vi "State of measurements func global.vi"(6 "Operation":T1(ring)=enum."Get", 9 "Active?":bool, 10 "Instruments in":refnum<class "Device.lvclass">[](array[class]), 11 "Measurement settings in":T4={"Measurements active"=FALSE, "Instruments"=[], "Save data settings"={"Save data"=TRUE, "Data Root Path"=path "", "File Prefix"="", "File Format"=enum."ASCII", "Save column names"=TRUE, "File Comments"="<Description of the current file>", "User/Prj"="<User Name/Project Description>"}, "Start time"=0}) -> (3 "Measurement settings out":T4={"Measurements active"=FALSE, "Instruments"=[], "Save data settings"={"Save data"=TRUE, "Data Root Path"=path "", "File Prefix"="", "File Format"=enum."ASCII", "Save column names"=TRUE, "File Comments"="<Description of the current file>", "User/Prj"="<User Name/Project Description>"}, "Start time"=0})   [LabVIEW 2015]
uses:
  Device/Device.lvclass
  File/Controls/Save data settings.ctl
  File/Controls/File formats.ctl
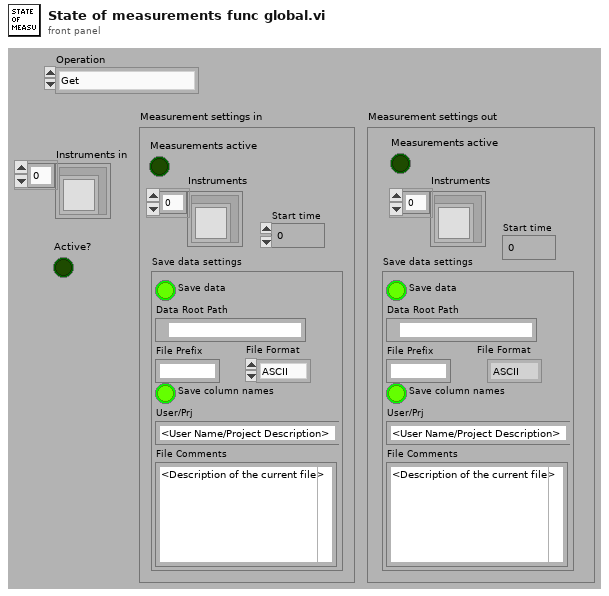
[diagram p1: front panel]
types:
  T1 = enum16{"Set", "Get", "Set Instruments", "Set active state"}
  T2 = typedef "Save data settings.ctl" = cluster{"Save data":bool, "Data Root Path":path, "File Prefix":string, "File Format":T3, "Save column names":bool, "File Comments":string, "User/Prj":string}
  T3 = typedef "File formats.ctl" = enum16{"TDMS", "ASCII", "BINARY"}
  T4 = cluster{"Measurements active":bool, "Instruments":refnum<class "Device.lvclass">[], "Save data settings":T2, "Start time":u32}
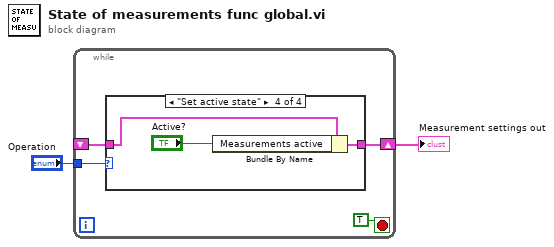
[diagram p0: block diagram]
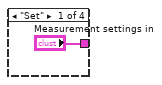
[diagram p2: hidden frame]
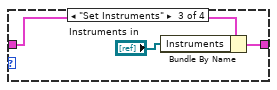
[diagram p4: hidden frame]
diagram:
  n1 = while {
    shift-right: [w5] -> w1
    shift-left: _ -> [w4]
    tunnel: "Operation" -> [w6]
    stop <- TRUE stop-if-true
    n2 = case shown="\"Set active state\"" w6 {
      tunnel: ["Measurement settings in" w8 w10 w13] -> w5
      tunnel: w4 -> [_ w8 w11 w14]
      frame "Set" {
      }
      frame "Get", Default {
      }
      frame "Set Instruments" {
        n3 = Bundle By Name(cluster=w11, "Instruments"="Instruments in") -> (w10:T4)
      }
      frame "Set active state" {
        n4 = Bundle By Name(cluster=w14, "Measurements active"="Active?") -> (w13:T4)
      }
    }
  }
  "Measurement settings out" <- w1
